vi "Read UI VI Ref.vi"(11 "Flex UI (Actor) in":refnum<class "Flex UI (Actor).lvclass">) -> (2 "UI VI Ref":refnum<class "MVC Subscription.lvclass">, 3 "Flex UI (Actor) out":refnum<class "Flex UI (Actor).lvclass">)   [LabVIEW 2016, in "Flex UI (Parent Actor).lvlib" / "Flex UI (Actor).lvclass"]
uses:
  Flex UI (Actor).lvclass
  <vilib>/East West Architects/MVC Subscription/Subscription/MVC Subscription.lvclass
  Flex UI (Actor).lvclass/Flex UI (Actor).ctl
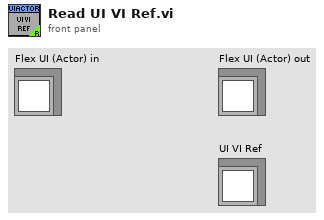
[diagram p1: front panel]
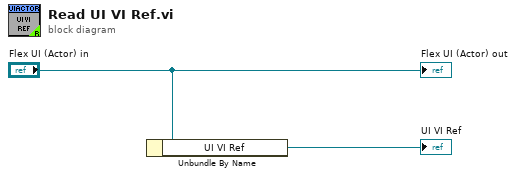
[diagram p0: block diagram]
diagram:
  n1 = Unbundle By Name("Flex UI (Actor) in") -> ("UI VI Ref"=→"UI VI Ref":refnum<class "MVC Subscription.lvclass">)
  "Flex UI (Actor) out" <- "Flex UI (Actor) in"
